vi "FPGA PWMs.vi"() -> ()   [LabVIEW 2025]
uses:
  FPGA IP/Types/PWM.Generate.Digital.Settings.ctl
  FPGA IP/Types/PWM.Measure.Digital.Settings.ctl
  FPGA IP/Types/PWM.Measure.Digital.Measurement.ctl
  <vilib>/Platform/TimedLoop/XDataNode/timing_clust.ctl
  <vilib>/Platform/TimedLoop/XDataNode/nitl_modes.ctl
  <vilib>/Platform/TimedLoop/XDataNode/wakeup.ctl
  <vilib>/rvi/Emulation/niFpgaGetClockAttributes.vi
  <vilib>/rvi/Emulation/niFpgaSctlEmulationGetInTimedLoop.vi
  <vilib>/rvi/Emulation/niFpgaEmulationReportErrorSimple.vi
  <vilib>/rvi/Emulation/niFpgaEmulationIsFPGAContextNoSignature.vi
  <vilib>/rvi/DataTransferAndStorage/Container/Common/niFpgaContainerGetUniqueNameForEmu.vi
  <vilib>/rvi/Memory/Memory_Emulation/niFpgaMemoryEmulationCacheClearOnFirstRun.vi
  <vilib>/rvi/Memory/Memory_Emulation/nirvimemoryEmulationManagerCache_MakeExclusive.vi
  <vilib>/rvi/Memory/Memory_Emulation/niFpgaMemoryEmulationValidateCache.vi
  <vilib>/rvi/Memory/Memory_Emulation/nirvimemoryEmulationManagerCache_InsertValue.vi
  <vilib>/Utility/error.llb/Clear Errors.vi
  <vilib>/rvi/Memory/Memory_Emulation/nirvimemoryEmulationManagerCache_ReleaseExclusive.vi
  <vilib>/rvi/Memory/Memory_Emulation/nirvimemoryEmulationManagerCache_GetValue.vi
  <vilib>/rvi/Memory/Memory_Emulation/nirvimemoryEmulationManagerCache_SetValue.vi
  <vilib>/rvi/Emulation/niFpgaProcessEmulError.vi
  <vilib>/rvi/eio/common/nirviEmuTemplateMethod_errors.vi
  <vilib>/rvi/Emulation/niFpgaCriticalErrorInLSC.vi
  <vilib>/rvi/DataTransferAndStorage/Container/XNode/niFpgaContainer.xnode
  <vilib>/rvi/DataTransferAndStorage/Register/Emulation/niFpgaRegisterEmulation.vi
  <vilib>/eio/EIONode/EIONode.xnode
  <vilib>/platform/TimedLoop/XDataNode/XDataNode.xnode
  FPGA IP/Speciality FPGA IO.lvlib
  <vilib>/Platform/TimedLoop/XDataNode/XDNodeRunTimeDep.lvlib
panel:
  out "Mod2 DI3 PWM Measurement":T1
  out "Mod2 DI0 PWM Measurement":T1
  in  "Mod2 DI3 PWM AcqSettings":T2={"ACTIVE EDGE"=TRUE, "TIMEOUT"=40000000}
  in  "Mod2 DI0 PWM AcqSettings":T2={"ACTIVE EDGE"=TRUE, "TIMEOUT"=40000000}
  in  "Mod2 PWM Gen Settings":T3={"ACTIVE EDGE"=TRUE, "ACTIVE TICKS"=0, "INACTIVE TICKS"=0}
  in  "Stop Fast PWM":bool
  in  "Stop Slow PWM":bool
  in  "Mod1 PWM Gen Settings":T3={"ACTIVE EDGE"=TRUE, "ACTIVE TICKS"=0, "INACTIVE TICKS"=0}
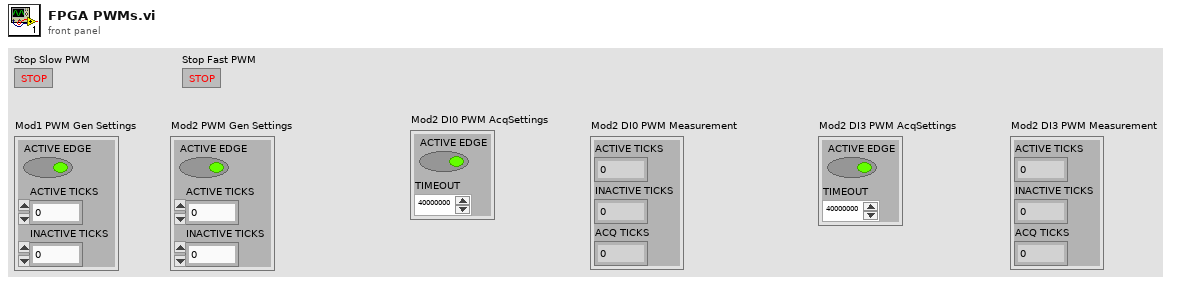
[diagram p1: front panel]
types:
  T1 = typedef "Speciality FPGA IO.lvlib/PWM.Measure.Digital.Measurement.ctl" = cluster{"ACTIVE TICKS":u32, "INACTIVE TICKS":u32, "ACQ TICKS":u32}
  T2 = typedef "Speciality FPGA IO.lvlib/PWM.Measure.Digital.Settings.ctl" = cluster{"ACTIVE EDGE":bool, "TIMEOUT":u32}
  T3 = typedef "Speciality FPGA IO.lvlib/PWM.Generate.Digital.Settings.ctl" = cluster{"ACTIVE EDGE":bool, "ACTIVE TICKS":u32, "INACTIVE TICKS":u32}
  T4 = typedef "XDNodeRunTimeDep.lvlib/timing_clust.ctl" = cluster{"Expected End [f-1]":u64, "Actual End [f-1]":u64, "Finished Late? [f-1]":bool, "Expected End [i-1]":u64, "Actual End [i-1]":u64, "Finished Late? [i-1]":bool, "Expected Start [i]":u64, "Actual Start [i]":u64, "Expected Start [f]":u64, "Actual Start [f]":u64, "Source Name":string, "Structure Name":string, "Period":i64, "Deadline":i64, "Offset":i64, "Start":i64, "Priority":i32, "Timeout":i32, "Mode":T5, "Wakeup Reason":T6, "Error":errorcluster, "Source Type":string, "Secondary Source Type":string, "Global End Time":u64, "Global Start Time":u64, "Frame Duration":u64, "Iteration Duration":u64, "Assigned CPU":i32, "I/O Scan Engine Mode":u32}
  T5 = typedef "XDNodeRunTimeDep.lvlib/nitl_modes.ctl" = enum32{"No Change", "Process missed periods, maintain original phase", "Discard missed periods, maintain original phase", "Process missed periods, ignore original phase", "Discard missed periods, ignore original phase"}
  T6 = typedef "XDNodeRunTimeDep.lvlib/wakeup.ctl" = enum32{"Normal", "Aborted", "Asynchronous wakeup", "Timing source error", "Timed loop error", "Timeout"}
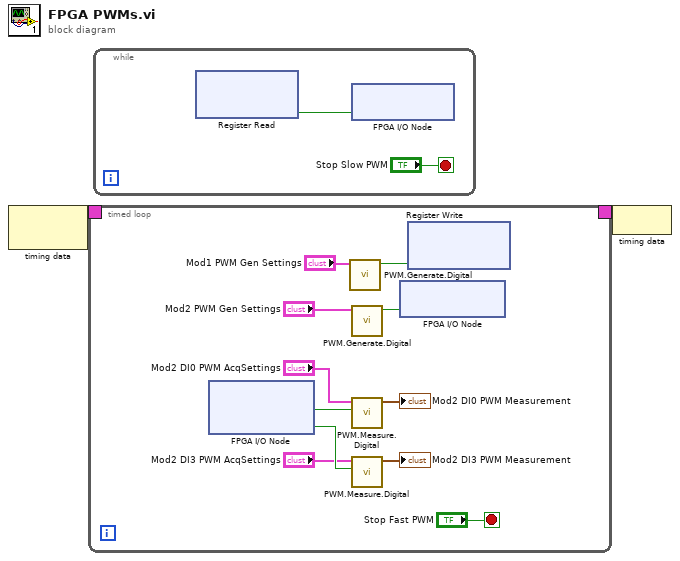
[diagram p0: block diagram]
diagram:
  n1 = node-c288() -> (w2:T4)  [unwired: 1 in]
  n2 = timed-loop {
    timing: w2 -> [_]
    timing-out: [_] -> w1
    stop <- "Stop Fast PWM" stop-if-true
    n3 = xnode "FPGA I/O Node"() -> ("Mod2/DIO0"=w10:bool, "Mod2/DIO3"=w9:bool)  [unwired: 2 in, 2 out]
    n4 = call "PWM.Generate.Digital.vi"("Settings"="Mod1 PWM Gen Settings") -> ("Output"=w3:bool)  [unwired: 10 in]
    n5 = call "PWM.Generate.Digital.vi"("Settings"="Mod2 PWM Gen Settings") -> ("Output"=w12:bool)  [unwired: 10 in]
    n6 = call "PWM.Measure.Digital.vi"("State"=w10, "Settings"="Mod2 DI0 PWM AcqSettings") -> ("Measurement"=→"Mod2 DI0 PWM Measurement":T1)  [unwired: 8 in, 1 out]
    n7 = call "PWM.Measure.Digital.vi"("State"=w9, "Settings"="Mod2 DI3 PWM AcqSettings") -> ("Measurement"=→"Mod2 DI3 PWM Measurement":T1)  [unwired: 8 in, 1 out]
    n8 = xnode "FPGA I/O Node"("Mod2/DIO4"=w12) -> ()  [unwired: 1 in, 1 out]
    n9 = xnode ("Register Write")("Data"=w3) -> ()  [unwired: 1 in, 1 out]
  }
  n10 = while {
    stop <- "Stop Slow PWM" stop-if-true
    n11 = xnode ("Register Read")() -> ("Data"=w16:bool)  [unwired: 1 in, 1 out]
    n12 = xnode "FPGA I/O Node"("Mod1/DO0"=w16) -> ()  [unwired: 1 in, 1 out]
  }
  n13 = node-c288(w1) -> ()
